vi "StringToU32(cast).vi"(1 "String":string) -> (0 "U32":u32)   [LabVIEW 2012]
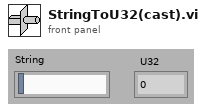
[diagram p1: front panel]
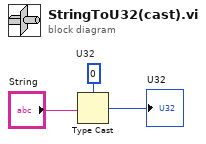
[diagram p0: block diagram]
diagram:
  w2 = u32 0  # U32
  n1 = Type Cast(type=w2, x="String") -> (*(type *) &x=→"U32":u32)
